vi "Create Type B.vi"(8 "error in (no error)":errorcluster, 10 "Barcode Content":string) -> (0 "error out":errorcluster, 3 "Barcode Reader out":refnum<class "Type B.lvclass">)   [LabVIEW 2020, in "Barcode Reader Second Iteration.lvlib" / "Type B.lvclass"]
uses:
  Type B.lvclass
  Type B.lvclass/Type B.ctl
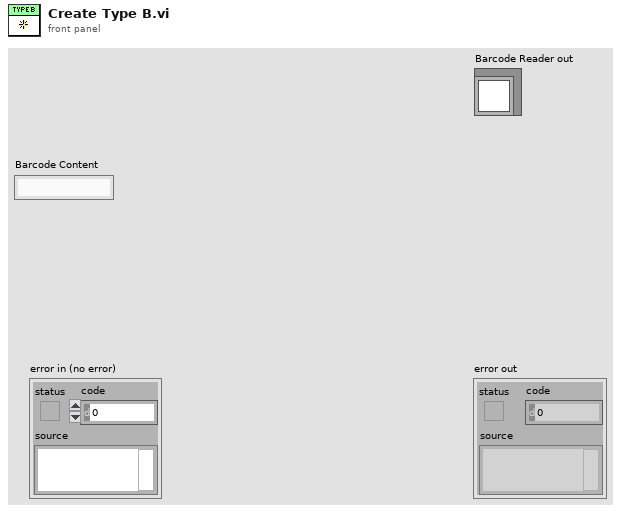
[diagram p1: front panel]
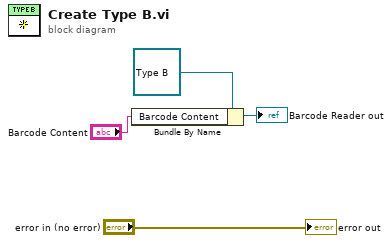
[diagram p0: block diagram]
diagram:
  n1 = Bundle By Name(cluster=refnum<class "Type B.lvclass"> refnum ("Barcode Reader in"), "Barcode Content"="Barcode Content") -> (→"Barcode Reader out":refnum<class "Type B.lvclass">)
  "error out" <- "error in (no error)"
